vi "Configure Spectral.vi"   [LabVIEW 2015, in "Tektronix 7000 Series.lvlib"]
doc: "This polymorphic VI configures the spectral responses of a mathematical waveform.\n\nThe tkdop7k Configure Spectral (Magnitude) VI configures the spectral magnitude.\n\nThe tkdop7k Configure Spectral (Phase) VI configures the spectral phase.\n\nThe tkdop7k Configure Spectral(Other) VI configures the spectral real and imaginary parts."
uses:
  <instrlib>/Tektronix 7000 Series/Tektronix 7000 Series.lvlib
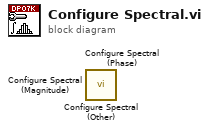
[diagram p0: block diagram]
diagram:
  n1 = call <instrlib>:"Configure Spectral (Other).vi"() -> ()  [unwired: 14 in, 2 out]
  n2 = call <instrlib>:"Configure Spectral (Phase).vi"() -> ()  [unwired: 14 in, 2 out]
  n3 = call <instrlib>:"Configure Spectral (Magnitude).vi"() -> ()  [unwired: 14 in, 2 out]
